vi "自定义双按钮对话框.vi"(8 "取消文本":string, 9 "确定文本":string, 10 "数值":i32=10, 11 "消息":string) -> (3 "输出":bool)   [LabVIEW 2016, in "数据传输系统-06.lvlib" / "update.lvlib"]
uses:
  update.lvlib
panel:
  in  "取消":bool
  out "计时":i32
  in  "确定":bool
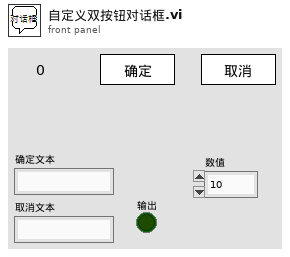
[diagram p1: front panel]
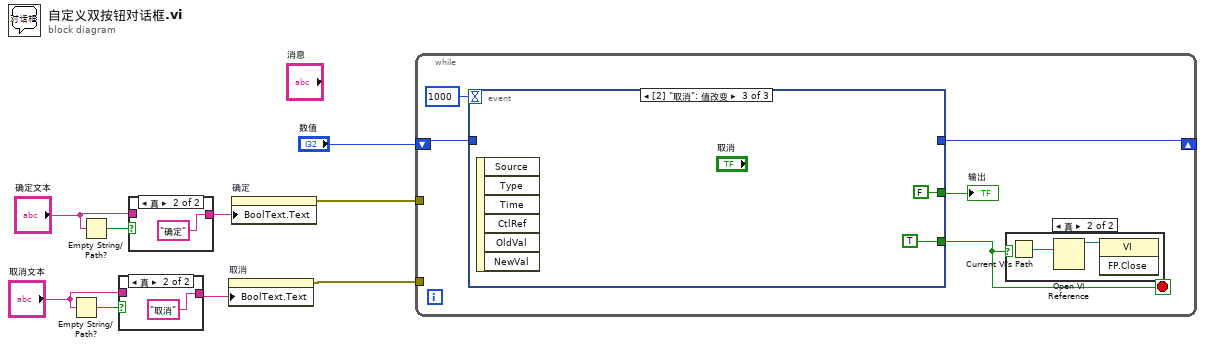
[diagram p0: block diagram]
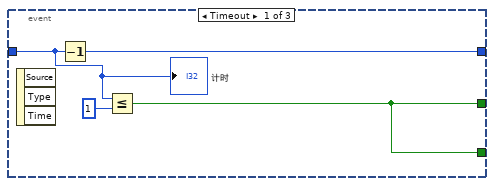
[diagram p3: hidden frame]
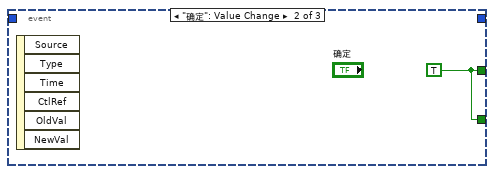
[diagram p4: hidden frame]
diagram:
  n1 = Empty String/Path?(string/path="取消文本") -> (empty?=w4:bool)
  n2 = Empty String/Path?(string/path="确定文本") -> (empty?=w7:bool)
  n3 = case shown="真" w4 {
    tunnel: [w10 "取消"] -> w2
    tunnel: "取消文本" -> [w10 _]
    frame False {
    }
    frame True {
    }
  }
  n4 = case shown="真" w7 {
    tunnel: [w12 "确定"] -> w6
    tunnel: "确定文本" -> [w12 _]
    frame False {
    }
    frame True {
    }
  }
  n5 = property on="取消" class="Bool"("BoolText.Text"=w2) -> (error out=w1:errorcluster)  [unwired: 2 in, 1 out]
  n6 = property on="确定" class="Bool"("BoolText.Text"=w6) -> (error out=w8:errorcluster)  [unwired: 2 in, 1 out]
  n7 = while {
    shift-right: [w18] -> _
    shift-left: "数值" -> [w17]
    tunnel: w8 -> [_]
    tunnel: w1 -> [_]
    stop <- w14 stop-if-true
    n8 = event shown="[2] \"取消\": 值改变" {
      selector: _ -> [_ _ _]
      dyn-events: _ -> [_ _ _]
      timeout: 1000 -> [_ _ _]
      tunnel: [w24 _ _] -> w18
      tunnel: w17 -> [w23 _ _]
      tunnel: [w21 w25 FALSE ("确定")] -> w15
      tunnel: [w21 w25 TRUE] -> w14
      event Timeout {
        n9 = event-data() -> ()  [unwired: 1 in, 3 out]
        n10 = Decrement(x=w23) -> (x-1=w24:i32)
        n11 = Less Or Equal?(x=w23, y=1) -> (x <= y?=w21:bool)
        "计时" <- w23
      }
      event "确定": Value Change {
        w25 = TRUE ("确定")
        n12 = event-data() -> ()  [unwired: 1 in, 6 out]
      }
      event "取消": Value Change {
        n13 = event-data() -> ()  [unwired: 1 in, 6 out]
      }
    }
    "输出" <- w15
    n14 = case shown="真" w14 {
      frame False {
      }
      frame True {
        n15 = Current VI's Path() -> (path=w20:path)
        n16 = Open VI Reference(vi path=w20) -> (vi reference=w19:refnum<vi>)  [unwired: 5 in, 1 out]
        n17 = invoke class="VI" method="FP.Close"(reference=w19) -> ()  [unwired: 2 in, 3 out]
      }
    }
  }
